vi "GetType.vi"(8 "error in (no error)":errorcluster, 11 "Configure TrigSlope Msg":refnum<class "Configure TrigSlope Msg.lvclass">) -> (0 "error out":errorcluster, 2 "Data Sample":variant, 3 "Configure TrigSlope Msg":refnum<class "Configure TrigSlope Msg.lvclass">)   [LabVIEW 2015, in "CS++MCS.lvlib" / "Configure TrigSlope Msg.lvclass"]
uses:
  Configure TrigSlope Msg.lvclass
  Configure TrigSlope Msg.lvclass/Configure TrigSlope Msg.ctl
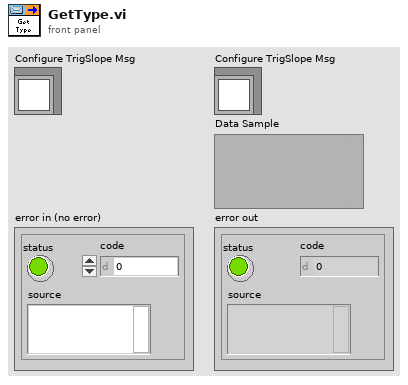
[diagram p1: front panel]
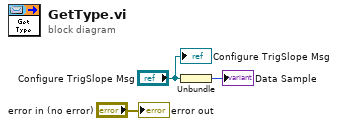
[diagram p0: block diagram]
diagram:
  n1 = Unbundle("Configure TrigSlope Msg") -> (→"Data Sample":u16)
  "error out" <- "error in (no error)"
  "Configure TrigSlope Msg" <- "Configure TrigSlope Msg"
